vi "DDS_Clock.vi"() -> ()   [LabVIEW 2016] (continued)
"f1 [Hz] CH0"=313000000.0}, {"total time[ms]"=53.29999999999911, "f1 [Hz] CH0"=313200000.00000006}, {"total time[ms]"=53.29999999999911, "f1 [Hz] CH0"=313200000.00000006}, {"total time[ms]"=53.349999999999106, "f1 [Hz] CH0"=313400000.00000006}, {"total time[ms]"=53.349999999999106, "f1 [Hz] CH0"=313400000.00000006}, {"total time[ms]"=53.3999999999991, "f1 [Hz] CH0"=313600000.0}, {"total time[ms]"=53.3999999999991, "f1 [Hz] CH0"=313600000.0}, {"total time[ms]"=53.4499999999991, "f1 [Hz] CH0"=313800000.0}, {"total time[ms]"=53.4499999999991, "f1 [Hz] CH0"=313800000.0}, {"total time[ms]"=53.4999999999991, "f1 [Hz] CH0"=314000000.0}, {"total time[ms]"=53.4999999999991, "f1 [Hz] CH0"=314000000.0}, {"total time[ms]"=53.549999999999095, "f1 [Hz] CH0"=314200000.0}, {"total time[ms]"=53.549999999999095, "f1 [Hz] CH0"=314200000.0}, {"total time[ms]"=53.59999999999909, "f1 [Hz] CH0"=314400000.0}, {"total time[ms]"=53.59999999999909, "f1 [Hz] CH0"=314400000.0}, {"total time[ms]"=53.64999999999909, "f1 [Hz] CH0"=314600000.00000006}, {"total time[ms]"=53.64999999999909, "f1 [Hz] CH0"=314600000.00000006}, {"total time[ms]"=53.699999999999086, "f1 [Hz] CH0"=314800000.00000006}, {"total time[ms]"=53.699999999999086, "f1 [Hz] CH0"=314800000.00000006}, {"total time[ms]"=53.74999999999908, "f1 [Hz] CH0"=315000000.0}, {"total time[ms]"=53.74999999999908, "f1 [Hz] CH0"=315000000.0}, {"total time[ms]"=53.79999999999908, "f1 [Hz] CH0"=315200000.00000006}, {"total time[ms]"=53.79999999999908, "f1 [Hz] CH0"=315200000.00000006}, {"total time[ms]"=53.84999999999908, "f1 [Hz] CH0"=315400000.0}, {"total time[ms]"=53.84999999999908, "f1 [Hz] CH0"=315400000.0}, {"total time[ms]"=53.899999999999075, "f1 [Hz] CH0"=315600000.0}, {"total time[ms]"=53.899999999999075, "f1 [Hz] CH0"=315600000.0}, {"total time[ms]"=53.94999999999907, "f1 [Hz] CH0"=315800000.0}, {"total time[ms]"=53.94999999999907, "f1 [Hz] CH0"=315800000.0}, {"total time[ms]"=53.99999999999907, "f1 [Hz] CH0"=316000000.0}, {"total time[ms]"=53.99999999999907, "f1 [Hz] CH0"=316000000.0}, {"total time[ms]"=54.049999999999066, "f1 [Hz] CH0"=316200000.00000006}, {"total time[ms]"=54.049999999999066, "f1 [Hz] CH0"=316200000.00000006}, {"total time[ms]"=54.09999999999906, "f1 [Hz] CH0"=316400000.0}, {"total time[ms]"=54.09999999999906, "f1 [Hz] CH0"=316400000.0}, {"total time[ms]"=54.14999999999906, "f1 [Hz] CH0"=316600000.00000006}, {"total time[ms]"=54.14999999999906, "f1 [Hz] CH0"=316600000.00000006}, {"total time[ms]"=54.19999999999906, "f1 [Hz] CH0"=316800000.00000006}, {"total time[ms]"=54.19999999999906, "f1 [Hz] CH0"=316800000.00000006}, {"total time[ms]"=54.249999999999055, "f1 [Hz] CH0"=317000000.0}, {"total time[ms]"=54.249999999999055, "f1 [Hz] CH0"=317000000.0}, {"total time[ms]"=54.29999999999905, "f1 [Hz] CH0"=317200000.0}, {"total time[ms]"=54.29999999999905, "f1 [Hz] CH0"=317200000.0}, {"total time[ms]"=54.34999999999905, "f1 [Hz] CH0"=317400000.0}, {"total time[ms]"=54.34999999999905, "f1 [Hz] CH0"=317400000.0}, {"total time[ms]"=54.39999999999905, "f1 [Hz] CH0"=317600000.00000006}, {"total time[ms]"=54.39999999999905, "f1 [Hz] CH0"=317600000.00000006}, {"total time[ms]"=54.449999999999044, "f1 [Hz] CH0"=317800000.0}, {"total time[ms]"=54.449999999999044, "f1 [Hz] CH0"=317800000.0}, {"total time[ms]"=54.49999999999904, "f1 [Hz] CH0"=318000000.0}, {"total time[ms]"=54.49999999999904, "f1 [Hz] CH0"=318000000.0}, {"total time[ms]"=54.54999999999904, "f1 [Hz] CH0"=318200000.00000006}, {"total time[ms]"=54.54999999999904, "f1 [Hz] CH0"=318200000.00000006}, {"total time[ms]"=54.599999999999035, "f1 [Hz] CH0"=318400000.00000006}, {"total time[ms]"=54.599999999999035, "f1 [Hz] CH0"=318400000.00000006}, {"total time[ms]"=54.64999999999903, "f1 [Hz] CH0"=318600000.0}, {"total time[ms]"=54.64999999999903, "f1 [Hz] CH0"=318600000.0}, {"total time[ms]"=54.69999999999903, "f1 [Hz] CH0"=318800000.0}, {"total time[ms]"=54.69999999999903, "f1 [Hz] CH0"=318800000.0}, {"total time[ms]"=54.74999999999903, "f1 [Hz] CH0"=319000000.0}, {"total time[ms]"=54.74999999999903, "f1 [Hz] CH0"=319000000.0}, {"total time[ms]"=54.799999999999024, "f1 [Hz] CH0"=319200000.0}, {"total time[ms]"=54.799999999999024, "f1 [Hz] CH0"=319200000.0}, {"total time[ms]"=54.84999999999902, "f1 [Hz] CH0"=319400000.0}, {"total time[ms]"=54.84999999999902, "f1 [Hz] CH0"=319400000.0}, {"total time[ms]"=54.89999999999902, "f1 [Hz] CH0"=319600000.00000006}, {"total time[ms]"=54.89999999999902, "f1 [Hz] CH0"=319600000.00000006}, {"total time[ms]"=54.949999999999015, "f1 [Hz] CH0"=319800000.00000006}, {"total time[ms]"=54.949999999999015, "f1 [Hz] CH0"=319800000.00000006}, {"total time[ms]"=54.99999999999901, "f1 [Hz] CH0"=320000000.0}, {"total time[ms]"=54.99999999999901, "f1 [Hz] CH0"=320000000.0}, {"total time[ms]"=55.04999999999901, "f1 [Hz] CH0"=319800000.0}, {"total time[ms]"=55.04999999999901, "f1 [Hz] CH0"=319800000.0}, {"total time[ms]"=55.09999999999901, "f1 [Hz] CH0"=319600000.0}, {"total time[ms]"=55.09999999999901, "f1 [Hz] CH0"=319600000.0}, {"total time[ms]"=55.149999999999004, "f1 [Hz] CH0"=319400000.0}, {"total time[ms]"=55.149999999999004, "f1 [Hz] CH0"=319400000.0}, {"total time[ms]"=55.199999999999, "f1 [Hz] CH0"=319200000.0}, {"total time[ms]"=55.199999999999, "f1 [Hz] CH0"=319200000.0}, {"total time[ms]"=55.249999999999, "f1 [Hz] CH0"=319000000.0}, {"total time[ms]"=55.249999999999, "f1 [Hz] CH0"=319000000.0}, {"total time[ms]"=55.299999999998995, "f1 [Hz] CH0"=318799999.99999994}, {"total time[ms]"=55.299999999998995, "f1 [Hz] CH0"=318799999.99999994}, {"total time[ms]"=55.34999999999899, "f1 [Hz] CH0"=318600000.0}, {"total time[ms]"=55.34999999999899, "f1 [Hz] CH0"=318600000.0}, {"total time[ms]"=55.39999999999899, "f1 [Hz] CH0"=318399999.99999994}, {"total time[ms]"=55.39999999999899, "f1 [Hz] CH0"=318399999.99999994}, {"total time[ms]"=55.44999999999899, "f1 [Hz] CH0"=318199999.99999994}, {"total time[ms]"=55.44999999999899, "f1 [Hz] CH0"=318199999.99999994}, {"total time[ms]"=55.499999999998984, "f1 [Hz] CH0"=318000000.0}, {"total time[ms]"=55.499999999998984, "f1 [Hz] CH0"=318000000.0}, {"total time[ms]"=55.54999999999898, "f1 [Hz] CH0"=317800000.0}, {"total time[ms]"=55.54999999999898, "f1 [Hz] CH0"=317800000.0}, {"total time[ms]"=55.59999999999898, "f1 [Hz] CH0"=317600000.0}, {"total time[ms]"=55.59999999999898, "f1 [Hz] CH0"=317600000.0}, {"total time[ms]"=55.649999999998975, "f1 [Hz] CH0"=317399999.99999994}, {"total time[ms]"=55.649999999998975, "f1 [Hz] CH0"=317399999.99999994}, {"total time[ms]"=55.69999999999897, "f1 [Hz] CH0"=317200000.0}, {"total time[ms]"=55.69999999999897, "f1 [Hz] CH0"=317200000.0}, {"total time[ms]"=55.74999999999897, "f1 [Hz] CH0"=317000000.0}, {"total time[ms]"=55.74999999999897, "f1 [Hz] CH0"=317000000.0}, {"total time[ms]"=55.79999999999897, "f1 [Hz] CH0"=316799999.99999994}, {"total time[ms]"=55.79999999999897, "f1 [Hz] CH0"=316799999.99999994}, {"total time[ms]"=55.849999999998964, "f1 [Hz] CH0"=316599999.99999994}, {"total time[ms]"=55.849999999998964, "f1 [Hz] CH0"=316599999.99999994}, {"total time[ms]"=55.89999999999896, "f1 [Hz] CH0"=316400000.0}, {"total time[ms]"=55.89999999999896, "f1 [Hz] CH0"=316400000.0}, {"total time[ms]"=55.94999999999896, "f1 [Hz] CH0"=316200000.0}, {"total time[ms]"=55.94999999999896, "f1 [Hz] CH0"=316200000.0}, {"total time[ms]"=55.999999999998956, "f1 [Hz] CH0"=316000000.0}, {"total time[ms]"=55.999999999998956, "f1 [Hz] CH0"=316000000.0}, {"total time[ms]"=56.04999999999895, "f1 [Hz] CH0"=315800000.0}, {"total time[ms]"=56.04999999999895, "f1 [Hz] CH0"=315800000.0}, {"total time[ms]"=56.09999999999895, "f1 [Hz] CH0"=315600000.0}, {"total time[ms]"=56.09999999999895, "f1 [Hz] CH0"=315600000.0}, {"total time[ms]"=56.14999999999895, "f1 [Hz] CH0"=315399999.99999994}, {"total time[ms]"=56.14999999999895, "f1 [Hz] CH0"=315399999.99999994}, {"total time[ms]"=56.199999999998944, "f1 [Hz] CH0"=315199999.99999994}, {"total time[ms]"=56.199999999998944, "f1 [Hz] CH0"=315199999.99999994}, {"total time[ms]"=56.24999999999894, "f1 [Hz] CH0"=315000000.0}, {"total time[ms]"=56.24999999999894, "f1 [Hz] CH0"=315000000.0}, {"total time[ms]"=56.29999999999894, "f1 [Hz] CH0"=314799999.99999994}, {"total time[ms]"=56.29999999999894, "f1 [Hz] CH0"=314799999.99999994}, {"total time[ms]"=56.349999999998936, "f1 [Hz] CH0"=314600000.0}, {"total time[ms]"=56.349999999998936, "f1 [Hz] CH0"=314600000.0}, {"total time[ms]"=56.39999999999893, "f1 [Hz] CH0"=314400000.0}, {"total time[ms]"=56.39999999999893, "f1 [Hz] CH0"=314400000.0}, {"total time[ms]"=56.44999999999893, "f1 [Hz] CH0"=314200000.0}, {"total time[ms]"=56.44999999999893, "f1 [Hz] CH0"=314200000.0}, {"total time[ms]"=56.49999999999893, "f1 [Hz] CH0"=314000000.0}, {"total time[ms]"=56.49999999999893, "f1 [Hz] CH0"=314000000.0}, {"total time[ms]"=56.549999999998924, "f1 [Hz] CH0"=313799999.99999994}, {"total time[ms]"=56.549999999998924, "f1 [Hz] CH0"=313799999.99999994}, {"total time[ms]"=56.59999999999892, "f1 [Hz] CH0"=313600000.0}, {"total time[ms]"=56.59999999999892, "f1 [Hz] CH0"=313600000.0}, {"total time[ms]"=56.64999999999892, "f1 [Hz] CH0"=313399999.99999994}, {"total time[ms]"=56.64999999999892, "f1 [Hz] CH0"=313399999.99999994}, {"total time[ms]"=56.699999999998916, "f1 [Hz] CH0"=313199999.99999994}, {"total time[ms]"=56.699999999998916, "f1 [Hz] CH0"=313199999.99999994}, {"total time[ms]"=56.74999999999891, "f1 [Hz] CH0"=313000000.0}, {"total time[ms]"=56.74999999999891, "f1 [Hz] CH0"=313000000.0}, {"total time[ms]"=56.79999999999891, "f1 [Hz] CH0"=312800000.0}, {"total time[ms]"=56.79999999999891, "f1 [Hz] CH0"=312800000.0}, {"total time[ms]"=56.84999999999891, "f1 [Hz] CH0"=312600000.0}, {"total time[ms]"=56.84999999999891, "f1 [Hz] CH0"=312600000.0}, {"total time[ms]"=56.899999999998904, "f1 [Hz] CH0"=312399999.99999994}, {"total time[ms]"=56.899999999998904, "f1 [Hz] CH0"=312399999.99999994}, {"total time[ms]"=56.9499999999989, "f1 [Hz] CH0"=312200000.0}, {"total time[ms]"=56.9499999999989, "f1 [Hz] CH0"=312200000.0}, {"total time[ms]"=56.9999999999989, "f1 [Hz] CH0"=312000000.0}, {"total time[ms]"=56.9999999999989, "f1 [Hz] CH0"=312000000.0}, {"total time[ms]"=57.049999999998896, "f1 [Hz] CH0"=311799999.99999994}, {"total time[ms]"=57.049999999998896, "f1 [Hz] CH0"=311799999.99999994}, {"total time[ms]"=57.09999999999889, "f1 [Hz] CH0"=311599999.99999994}, {"total time[ms]"=57.09999999999889, "f1 [Hz] CH0"=311599999.99999994}, {"total time[ms]"=57.14999999999889, "f1 [Hz] CH0"=311400000.0}, {"total time[ms]"=57.14999999999889, "f1 [Hz] CH0"=311400000.0}, {"total time[ms]"=57.19999999999889, "f1 [Hz] CH0"=311200000.0}, {"total time[ms]"=57.19999999999889, "f1 [Hz] CH0"=311200000.0}, {"total time[ms]"=57.249999999998884, "f1 [Hz] CH0"=311000000.0}, {"total time[ms]"=57.249999999998884, "f1 [Hz] CH0"=311000000.0}, {"total time[ms]"=57.29999999999888, "f1 [Hz] CH0"=310800000.0}, {"total time[ms]"=57.29999999999888, "f1 [Hz] CH0"=310800000.0}, {"total time[ms]"=57.34999999999888, "f1 [Hz] CH0"=310600000.0}, {"total time[ms]"=57.34999999999888, "f1 [Hz] CH0"=310600000.0}, {"total time[ms]"=57.399999999998876, "f1 [Hz] CH0"=310399999.99999994}, {"total time[ms]"=57.399999999998876, "f1 [Hz] CH0"=310399999.99999994}, {"total time[ms]"=57.44999999999887, "f1 [Hz] CH0"=310199999.99999994}, {"total time[ms]"=57.44999999999887, "f1 [Hz] CH0"=310199999.99999994}, {"total time[ms]"=57.49999999999887, "f1 [Hz] CH0"=310000000.0}, {"total time[ms]"=57.49999999999887, "f1 [Hz] CH0"=310000000.0}, {"total time[ms]"=57.54999999999887, "f1 [Hz] CH0"=309799999.99999994}, {"total time[ms]"=57.54999999999887, "f1 [Hz] CH0"=309799999.99999994}, {"total time[ms]"=57.599999999998865, "f1 [Hz] CH0"=309600000.0}, {"total time[ms]"=57.599999999998865, "f1 [Hz] CH0"=309600000.0}, {"total time[ms]"=57.64999999999886, "f1 [Hz] CH0"=309400000.0}, {"total time[ms]"=57.64999999999886, "f1 [Hz] CH0"=309400000.0}, {"total time[ms]"=57.69999999999886, "f1 [Hz] CH0"=309200000.0}, {"total time[ms]"=57.69999999999886, "f1 [Hz] CH0"=309200000.0}, {"total time[ms]"=57.749999999998856, "f1 [Hz] CH0"=309000000.0}, {"total time[ms]"=57.749999999998856, "f1 [Hz] CH0"=309000000.0}, {"total time[ms]"=57.79999999999885, "f1 [Hz] CH0"=308799999.99999994}, {"total time[ms]"=57.79999999999885, "f1 [Hz] CH0"=308799999.99999994}, {"total time[ms]"=57.84999999999885, "f1 [Hz] CH0"=308600000.0}, {"total time[ms]"=57.84999999999885, "f1 [Hz] CH0"=308600000.0}, {"total time[ms]"=57.89999999999885, "f1 [Hz] CH0"=308399999.99999994}, {"total time[ms]"=57.89999999999885, "f1 [Hz] CH0"=308399999.99999994}, {"total time[ms]"=57.949999999998845, "f1 [Hz] CH0"=308199999.99999994}, {"total time[ms]"=57.949999999998845, "f1 [Hz] CH0"=308199999.99999994}, {"total time[ms]"=57.99999999999884, "f1 [Hz] CH0"=308000000.0}, {"total time[ms]"=57.99999999999884, "f1 [Hz] CH0"=308000000.0}, {"total time[ms]"=58.04999999999884, "f1 [Hz] CH0"=307800000.0}, {"total time[ms]"=58.04999999999884, "f1 [Hz] CH0"=307800000.0}, {"total time[ms]"=58.099999999998836, "f1 [Hz] CH0"=307600000.0}, {"total time[ms]"=58.099999999998836, "f1 [Hz] CH0"=307600000.0}, {"total time[ms]"=58.14999999999883, "f1 [Hz] CH0"=307399999.99999994}, {"total time[ms]"=58.14999999999883, "f1 [Hz] CH0"=307399999.99999994}, {"total time[ms]"=58.19999999999883, "f1 [Hz] CH0"=307200000.0}, {"total time[ms]"=58.19999999999883, "f1 [Hz] CH0"=307200000.0}, {"total time[ms]"=58.24999999999883, "f1 [Hz] CH0"=307000000.0}, {"total time[ms]"=58.24999999999883, "f1 [Hz] CH0"=307000000.0}, {"total time[ms]"=58.299999999998825, "f1 [Hz] CH0"=306799999.99999994}, {"total time[ms]"=58.299999999998825, "f1 [Hz] CH0"=306799999.99999994}, {"total time[ms]"=58.34999999999882, "f1 [Hz] CH0"=306599999.99999994}, {"total time[ms]"=58.34999999999882, "f1 [Hz] CH0"=306599999.99999994}, {"total time[ms]"=58.39999999999882, "f1 [Hz] CH0"=306400000.0}, {"total time[ms]"=58.39999999999882, "f1 [Hz] CH0"=306400000.0}, {"total time[ms]"=58.449999999998816, "f1 [Hz] CH0"=306200000.0}, {"total time[ms]"=58.449999999998816, "f1 [Hz] CH0"=306200000.0}, {"total time[ms]"=58.49999999999881, "f1 [Hz] CH0"=306000000.0}, {"total time[ms]"=58.49999999999881, "f1 [Hz] CH0"=306000000.0}, {"total time[ms]"=58.54999999999881, "f1 [Hz] CH0"=305800000.0}, {"total time[ms]"=58.54999999999881, "f1 [Hz] CH0"=305800000.0}, {"total time[ms]"=58.59999999999881, "f1 [Hz] CH0"=305600000.0}, {"total time[ms]"=58.59999999999881, "f1 [Hz] CH0"=305600000.0}, {"total time[ms]"=58.649999999998805, "f1 [Hz] CH0"=305399999.99999994}, {"total time[ms]"=58.649999999998805, "f1 [Hz] CH0"=305399999.99999994}, {"total time[ms]"=58.6999999999988, "f1 [Hz] CH0"=305199999.99999994}, {"total time[ms]"=58.6999999999988, "f1 [Hz] CH0"=305199999.99999994}, {"total time[ms]"=58.7499999999988, "f1 [Hz] CH0"=305000000.0}, {"total time[ms]"=58.7499999999988, "f1 [Hz] CH0"=305000000.0}, {"total time[ms]"=58.799999999998796, "f1 [Hz] CH0"=304799999.99999994}, {"total time[ms]"=58.799999999998796, "f1 [Hz] CH0"=304799999.99999994}, {"total time[ms]"=58.84999999999879, "f1 [Hz] CH0"=304600000.0}, {"total time[ms]"=58.84999999999879, "f1 [Hz] CH0"=304600000.0}, {"total time[ms]"=58.89999999999879, "f1 [Hz] CH0"=304400000.0}, {"total time[ms]"=58.89999999999879, "f1 [Hz] CH0"=304400000.0}, {"total time[ms]"=58.94999999999879, "f1 [Hz] CH0"=304200000.0}, {"total time[ms]"=58.94999999999879, "f1 [Hz] CH0"=304200000.0}, {"total time[ms]"=58.999999999998785, "f1 [Hz] CH0"=304000000.0}, {"total time[ms]"=58.999999999998785, "f1 [Hz] CH0"=304000000.0}, {"total time[ms]"=59.04999999999878, "f1 [Hz] CH0"=303799999.99999994}, {"total time[ms]"=59.04999999999878, "f1 [Hz] CH0"=303799999.99999994}, {"total time[ms]"=59.09999999999878, "f1 [Hz] CH0"=303600000.0}, {"total time[ms]"=59.09999999999878, "f1 [Hz] CH0"=303600000.0}, {"total time[ms]"=59.149999999998776, "f1 [Hz] CH0"=303399999.99999994}, {"total time[ms]"=59.149999999998776, "f1 [Hz] CH0"=303399999.99999994}, {"total time[ms]"=59.199999999998774, "f1 [Hz] CH0"=303199999.99999994}, {"total time[ms]"=59.199999999998774, "f1 [Hz] CH0"=303199999.99999994}, {"total time[ms]"=59.24999999999877, "f1 [Hz] CH0"=303000000.0}, {"total time[ms]"=59.24999999999877, "f1 [Hz] CH0"=303000000.0}, {"total time[ms]"=59.29999999999877, "f1 [Hz] CH0"=302800000.0}, {"total time[ms]"=59.29999999999877, "f1 [Hz] CH0"=302800000.0}, {"total time[ms]"=59.349999999998765, "f1 [Hz] CH0"=302600000.0}, {"total time[ms]"=59.349999999998765, "f1 [Hz] CH0"=302600000.0}, {"total time[ms]"=59.39999999999876, "f1 [Hz] CH0"=302399999.99999994}, {"total time[ms]"=59.39999999999876, "f1 [Hz] CH0"=302399999.99999994}, {"total time[ms]"=59.44999999999876, "f1 [Hz] CH0"=302200000.0}, {"total time[ms]"=59.44999999999876, "f1 [Hz] CH0"=302200000.0}, {"total time[ms]"=59.49999999999876, "f1 [Hz] CH0"=302000000.0}, {"total time[ms]"=59.49999999999876, "f1 [Hz] CH0"=302000000.0}, {"total time[ms]"=59.549999999998754, "f1 [Hz] CH0"=301799999.99999994}, {"total time[ms]"=59.549999999998754, "f1 [Hz] CH0"=301799999.99999994}, {"total time[ms]"=59.59999999999875, "f1 [Hz] CH0"=301599999.99999994}, {"total time[ms]"=59.59999999999875, "f1 [Hz] CH0"=301599999.99999994}, {"total time[ms]"=59.64999999999875, "f1 [Hz] CH0"=301400000.0}, {"total time[ms]"=59.64999999999875, "f1 [Hz] CH0"=301400000.0}, {"total time[ms]"=59.699999999998745, "f1 [Hz] CH0"=301200000.0}, {"total time[ms]"=59.699999999998745, "f1 [Hz] CH0"=301200000.0}, {"total time[ms]"=59.74999999999874, "f1 [Hz] CH0"=301000000.0}, {"total time[ms]"=59.74999999999874, "f1 [Hz] CH0"=301000000.0}, {"total time[ms]"=59.79999999999874, "f1 [Hz] CH0"=300800000.0}, {"total time[ms]"=59.79999999999874, "f1 [Hz] CH0"=300800000.0}, {"total time[ms]"=59.84999999999874, "f1 [Hz] CH0"=300600000.0}, {"total time[ms]"=59.84999999999874, "f1 [Hz] CH0"=300600000.0}, {"total time[ms]"=59.899999999998734, "f1 [Hz] CH0"=300399999.99999994}, {"total time[ms]"=59.899999999998734, "f1 [Hz] CH0"=300399999.99999994}, {"total time[ms]"=59.94999999999873, "f1 [Hz] CH0"=300199999.99999994}, {"total time[ms]"=59.94999999999873, "f1 [Hz] CH0"=300199999.99999994}, {"total time[ms]"=59.99999999999873, "f1 [Hz] CH0"=300000000.0}, {"total time[ms]"=59.99999999999873, "f1 [Hz] CH0"=300000000.0}, {"total time[ms]"=60.049999999998725, "f1 [Hz] CH0"=300200000.00000006}, {"total time[ms]"=60.049999999998725, "f1 [Hz] CH0"=300200000.00000006}, {"total time[ms]"=60.09999999999872, "f1 [Hz] CH0"=300400000.0}, {"total time[ms]"=60.09999999999872, "f1 [Hz] CH0"=300400000.0}, {"total time[ms]"=60.14999999999872, "f1 [Hz] CH0"=300600000.0}, {"total time[ms]"=60.14999999999872, "f1 [Hz] CH0"=300600000.0}, {"total time[ms]"=60.19999999999872, "f1 [Hz] CH0"=300800000.0}, {"total time[ms]"=60.19999999999872, "f1 [Hz] CH0"=300800000.0}, {"total time[ms]"=60.249999999998714, "f1 [Hz] CH0"=301000000.0}, {"total time[ms]"=60.249999999998714, "f1 [Hz] CH0"=301000000.0}, {"total time[ms]"=60.29999999999871, "f1 [Hz] CH0"=301200000.00000006}, {"total time[ms]"=60.29999999999871, "f1 [Hz] CH0"=301200000.00000006}, {"total time[ms]"=60.34999999999871, "f1 [Hz] CH0"=301400000.0}, {"total time[ms]"=60.34999999999871, "f1 [Hz] CH0"=301400000.0}, {"total time[ms]"=60.399999999998705, "f1 [Hz] CH0"=301600000.00000006}, {"total time[ms]"=60.399999999998705, "f1 [Hz] CH0"=301600000.00000006}, {"total time[ms]"=60.4499999999987, "f1 [Hz] CH0"=301800000.00000006}, {"total time[ms]"=60.4499999999987, "f1 [Hz] CH0"=301800000.00000006}, {"total time[ms]"=60.4999999999987, "f1 [Hz] CH0"=302000000.0}, {"total time[ms]"=60.4999999999987, "f1 [Hz] CH0"=302000000.0}, {"total time[ms]"=60.5499999999987, "f1 [Hz] CH0"=302200000.0}, {"total time[ms]"=60.5499999999987, "f1 [Hz] CH0"=302200000.0}, {"total time[ms]"=60.599999999998694, "f1 [Hz] CH0"=302400000.0}, {"total time[ms]"=60.599999999998694, "f1 [Hz] CH0"=302400000.0}, {"total time[ms]"=60.64999999999869, "f1 [Hz] CH0"=302600000.00000006}, 
